vi "Query Device Name.vi"(8 "error in (no error)":errorcluster, 11 "VISA resource name":refnum<visa-resource-name>) -> (0 "error out":errorcluster, 2 "Device Name":string, 3 "VISA resource name out":refnum<visa-resource-name>)   [LabVIEW 2014, in "Associated Research SC6540.lvlib"]
doc: "Query the Device Name configured in the instrument"
uses:
  <instrlib>/Associated Research SC6540/Associated Research SC6540.lvlib
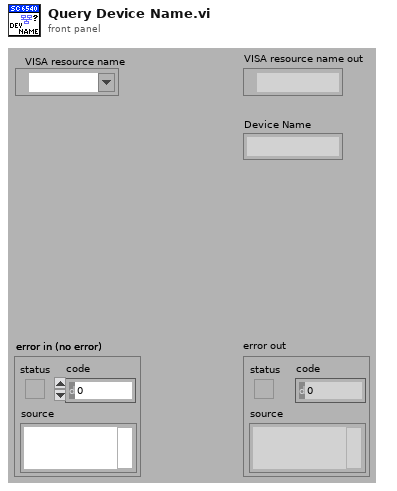
[diagram p1: front panel]
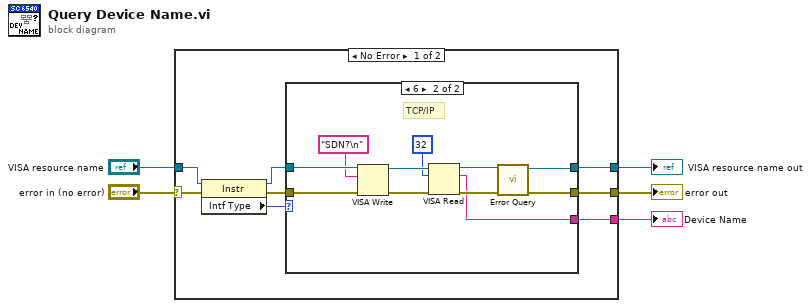
[diagram p0: block diagram]
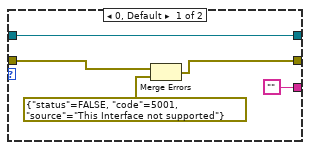
[diagram p2: hidden frame]
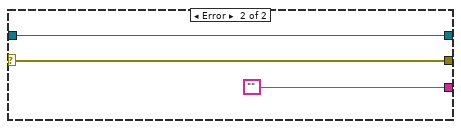
[diagram p3: hidden frame]
diagram:
  n1 = case shown="No Error" "error in (no error)" {
    selector: "error in (no error)" -> [w11 w32]
    tunnel: "VISA resource name" -> [w8 w31]
    tunnel: [w13 w31] -> w3
    tunnel: [w12 w32] -> w2
    tunnel: [w10 ""] -> w1
    frame No Error {
      n2 = property class="Instr"(reference=w8, error in=w11) -> (reference out=w7:refnum<visa-resource-name>, error out=w9:errorcluster, "Intf Type"=w6:u16)
      n3 = case shown="6" w6 {
        tunnel: w7 -> [w14 w29]
        tunnel: [w14 w28] -> w13
        tunnel: [w16 w27] -> w12
        tunnel: w9 -> [w17 w25]
        tunnel: ["" w19] -> w10
        frame 0, Default {
          n4 = Merge Errors(w17, errorcluster {"status"=FALSE, "code"=5001, "source"="This Interface not supported"} ("error in 2 (no error)")) -> (w16:errorcluster)
        }
        frame 6 {
          # "TCP/IP"
          n5 = VISA Write(VISA resource name=w29, write buffer="SDN?\n" ("Command to Send"), error in (no error)=w25) -> (VISA resource name out=w23:refnum<visa-resource-name>, error out=w24:errorcluster)  [unwired: 1 out]
          n6 = VISA Read(VISA resource name=w23, byte count=u32 32, error in (no error)=w24) -> (VISA resource name out=w22:refnum<visa-resource-name>, read buffer=w19:string, error out=w21:errorcluster)  [unwired: 1 out]
          n7 = call <instrlib>:"Error Query.vi"("error in (no error)"=w21, "VISA resource name"=w22) -> ("error out"=w27:errorcluster, "VISA resource name out"=w28:refnum<visa-resource-name>)  [unwired: 6 in, 2 out]
        }
      }
    }
    frame Error {
    }
  }
  "error out" <- w2
  "VISA resource name out" <- w3
  "Device Name" <- w1
